vi "GF_InsertChannelInformation.vi"(0 "VISA resource name":refnum<visa-resource-name>, 1 "Channel Name":string, 5 "Waveform In":waveform(dbl), 7 "Source (0: Channel 1)":u16(ring) items=["Channel 1", "Channel 2", "Channel 3", "Channel 4", "Math"], 9 "Timeout (10000 ms)":u32=10000, 11 "error in (no error)":errorcluster, 12 "Timing Info":cluster{"Name":string, "Value":string}[](array[cluster])) -> (4 "VISA resource name out":refnum<visa-resource-name>, 6 "waveform out":waveform(dbl), 15 "error out":errorcluster)   [LabVIEW 2020]
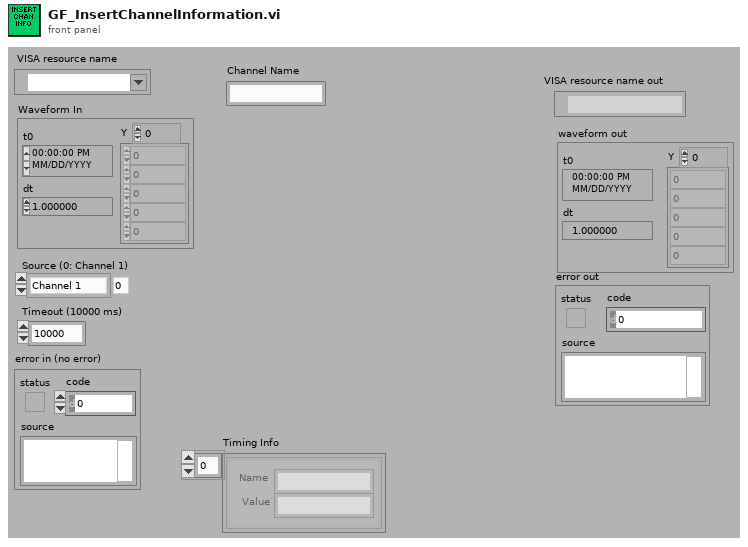
[diagram p1: front panel]
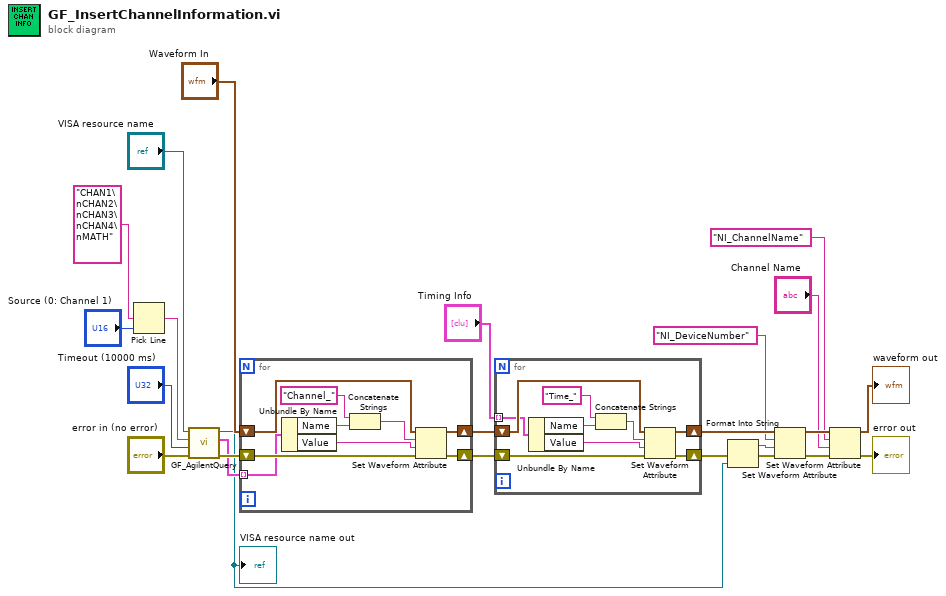
[diagram p0: block diagram]
diagram:
  n1 = Pick Line(multi-line string="CHAN1\nCHAN2\nCHAN3\nCHAN4\nMATH", line index="Source (0: Channel 1)") -> (output string=w19:string)  [unwired: 1 in]
  n2 = call "GF_AgilentQuery.vi"("error in (no error)"="error in (no error)", "Timeout"="Timeout (10000 ms)", "Query"=w19, "Session In"="VISA resource name") -> ("error out"=w18:errorcluster, "Token Array 2"=w16:cluster{"Name":string, "Value":string}[], "Session out"=w10:refnum<visa-resource-name>)  [unwired: 4 in]
  "VISA resource name out" <- w10
  n3 = for {
    shift-right: [w33] -> w14
    shift-left: w18 -> [w32]
    shift-right: [w30] -> w15
    shift-left: "Waveform In" -> [w31]
    tunnel: w16 -> [w29] mode=indexing
    n4 = Unbundle By Name(w29) -> ("Name"=w26:string, "Value"=w28:string)
    n5 = Concatenate Strings("Channel_", w26) -> (w25:string)
    n6 = Set Waveform Attribute(4:w32, 5:w28, 6:w25, 7:w31) -> (0:w33:errorcluster, 3:w30:waveform(dbl))  [unwired: 1 out]
  }
  n7 = for {
    shift-right: [w42] -> w8
    shift-left: w14 -> [w41]
    shift-right: [w39] -> w12
    shift-left: w15 -> [w40]
    tunnel: "Timing Info" -> [w38] mode=indexing
    n8 = Unbundle By Name(w38) -> ("Name"=w35:string, "Value"=w37:string)
    n9 = Concatenate Strings("Time_", w35) -> (w34:string)
    n10 = Set Waveform Attribute(4:w41, 5:w37, 6:w34, 7:w40) -> (0:w42:errorcluster, 3:w39:waveform(dbl))  [unwired: 1 out]
  }
  n11 = Format Into String(error in=w8, w10) -> (resulting string=w9:string, error out=w7:errorcluster)  [unwired: 2 in]
  n12 = Set Waveform Attribute(4:w7, 5:w9, 6:"NI_DeviceNumber", 7:w12) -> (0:w3:errorcluster, 3:w6:waveform(dbl))  [unwired: 1 out]
  n13 = Set Waveform Attribute(4:w3, 5:"Channel Name", 6:"NI_ChannelName" ("name"), 7:w6) -> (0:→"error out":errorcluster, 3:→"waveform out":waveform(dbl))  [unwired: 1 out]
